vi "Tx Channel Config Page.vi"(8 "error in (no error)":errorcluster, 11 "Node Ptr":T1 format="%.0x") -> (0 "error out":errorcluster)   [LabVIEW 2019, in "UDP-Custom-Device System Explorer.lvlib"]
uses:
  UDP-Custom-Device System Explorer.lvlib
  <vilib>/NI VeriStand/Custom Device API/Custom Device Item Ref.ctl
  Shared/Constants.vi
  <vilib>/NI VeriStand/Custom Device API/Set Item Property (Boolean).vi
  <vilib>/NI VeriStand/Custom Device API/Set Item Property (U32).vi
  <vilib>/NI VeriStand/Custom Device API/Custom Device API.lvlib
  Property Accessors/Shared Channel Accessors.lvlib
  <vilib>/NI VeriStand/Custom Device Tools/Custom Device Utility Library/Custom Device Utility Library.lvlib
  Shared/UDP-Custom-Device Shared.lvlib
panel:
  in  "Append To Channels":bool
  in  "Instances To Create":u32=1 min=1 step=1
  out "Imported Channel Configuration":i32[](listbox) caption="Channels"
  in  "Channel Configuration File":path
  in  "Description":string
  out "Name":string
  in  "SHDocVw.IWebBrowser":refnum<k7>(container)
  in  "General Header":cluster{"Section Name":string}={"Section Name"="Channel Configuration"}
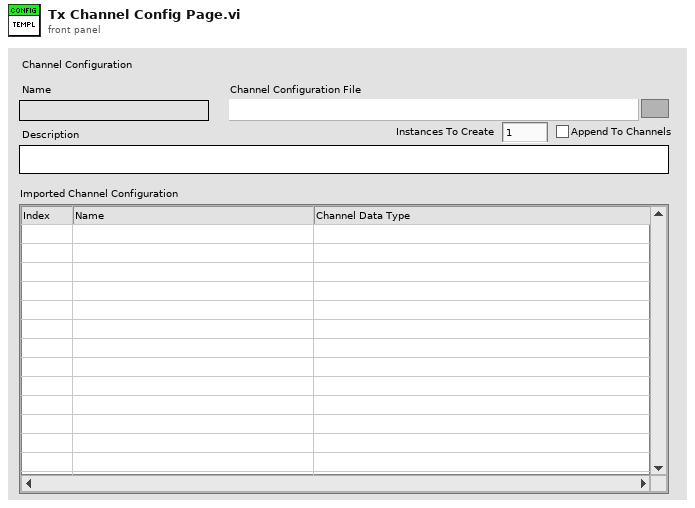
[diagram p1: front panel]
types:
  T1 = typedef "Custom Device API.lvlib/Custom Device Item Ref.ctl" = u64
  T2 = typedef "Custom Device API.lvlib/Custom Device Commands.ctl" = enum16{"Default", "Item renamed", "Shutdown", "Dynamic button pressed"}
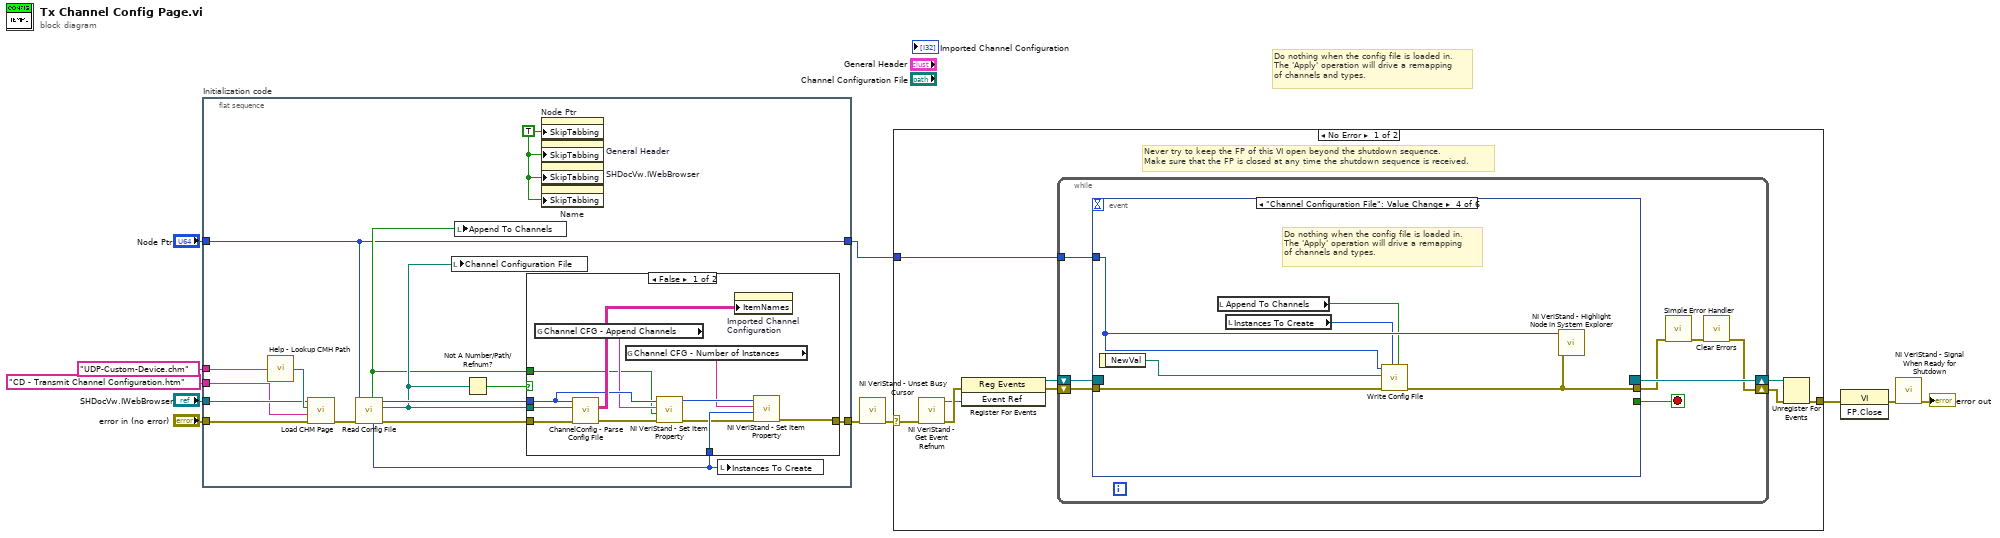
[diagram p0: block diagram]
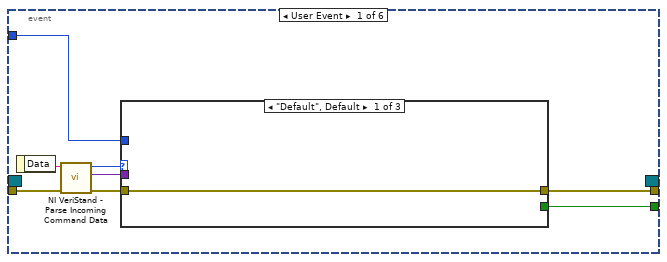
[diagram p3: hidden frame]
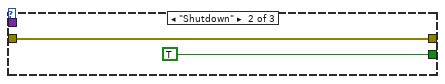
[diagram p4: hidden frame]
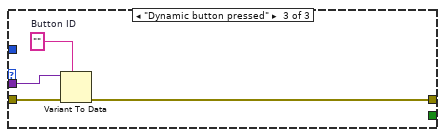
[diagram p5: hidden frame]
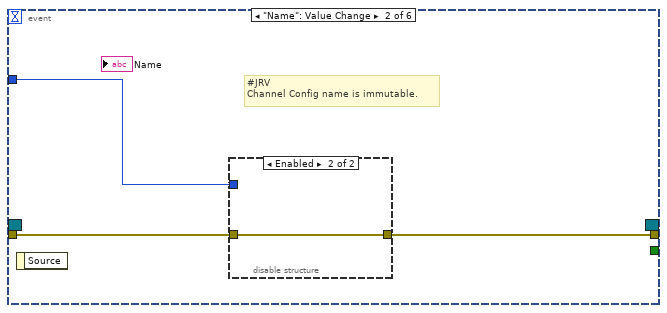
[diagram p6: hidden frame]
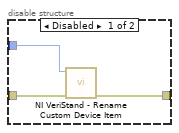
[diagram p7: hidden frame]
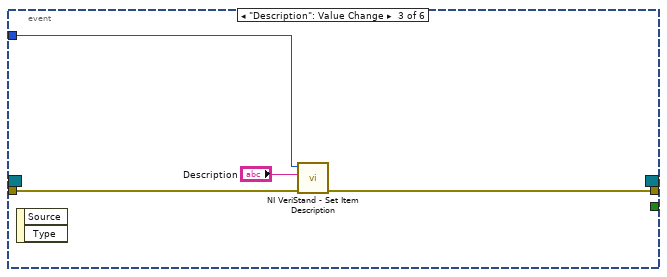
[diagram p8: hidden frame]
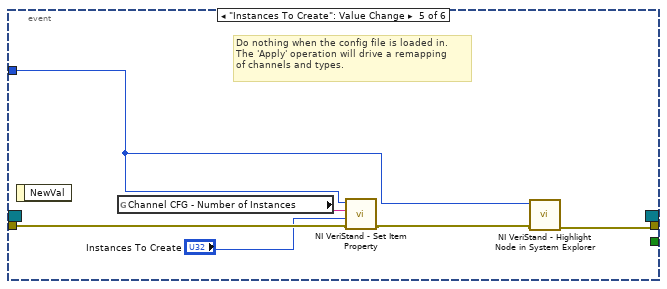
[diagram p9: hidden frame]
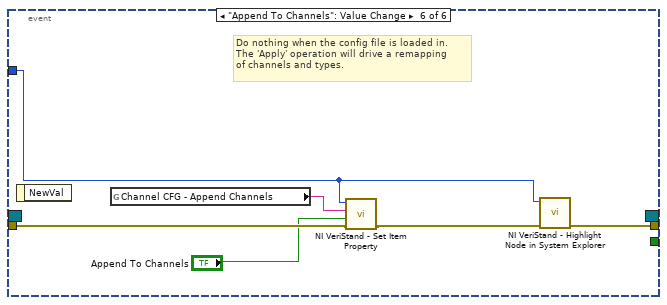
[diagram p10: hidden frame]
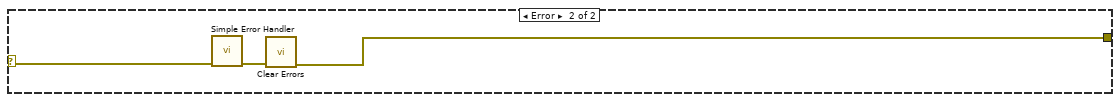
[diagram p11: hidden frame]
diagram:
  # "Do nothing when the config file is loaded in.\nThe 'Apply' operation will drive a remapping\nof channels and types."
  n1 = flat-sequence "Initialization code" {
    tunnel: "error in (no error)" -> [w25]
    tunnel: "Node Ptr" -> [w12]
    tunnel: [w16] -> w7
    tunnel: [w12] -> w4
    tunnel: "SHDocVw.IWebBrowser" -> [w24]
    tunnel: "CD - Transmit Channel Configuration.htm" ("CD_CHM_Section") -> [w22]
    tunnel: "UDP-Custom-Device.chm" ("CD_CHM_FileName") -> [w23]
    frame #0 {
      w15 = TRUE ("Skip When Tabbing")
      n2 = call "Help - Lookup CMH Path.vi"("Main CMH File"=w23) -> ("Compiled CMH Path"=w26:path)
      n3 = call <vilib>:"Load CHM Page.vi"("error in (no error)"=w25, "HTML File"=w22, "Compiled CHM Path"=w26, "Web Browser Reference"=w24) -> ("error out"=w21:errorcluster)  [unwired: 7 in]
      n4 = call "Read Config File.vi"("error in (no error)"=w21, "Node Ptr"=w12) -> ("error out"=w20:errorcluster, "Config File"=w17:path, "Node Ptr out"=w18:T1, "NumberOfInstances"=w13:u32, "AppendToChannels"=w14:bool)  [unwired: 5 in]
      n5 = local write "Channel Configuration File"(w17) -> ()
      n6 = local write "Append To Channels"(w14) -> ()
      n7 = Not A Number/Path/Refnum?(number/path/refnum=w17) -> (NaN/Path/Refnum?=w19:bool)
      n8 = case shown="False" w19 {
        tunnel: w20 -> [w38 w39]
        tunnel: w18 -> [w34 _]
        tunnel: w17 -> [w37 _]
        tunnel: [w27 w39] -> w16
        tunnel: w14 -> [w31 _]
        tunnel: w13 -> [w30 _]
        frame False {
          n9 = global read "Constants.vi" "Channel CFG - Append Channels"() -> (w33:string)
          n10 = call "ChannelConfig - Parse Config File.vi"("error in (no error)"=w38, "Config Path"=w37, "Node Ptr"=w34) -> ("error out"=w29:errorcluster, "Channel Configuration"=w36:string[][])  [unwired: 6 in, 1 out]
          n11 = global read "Constants.vi" "Channel CFG - Number of Instances"() -> (w32:string)
          n12 = call-poly <vilib>:"NI VeriStand - Set Item Property.vi"("error in (no error)"=w29, "Value"=w31, "Property Name"=w33, "Item Ref in"=w34) -> ("error out"=w28:errorcluster, "Item Ref out"=w35:T1)  [unwired: 5 in, 1 out]
          n13 = property on="Imported Channel Configuration" class="MCListbox (strict)"("ItemNames"=w36) -> ()  [unwired: 2 in, 2 out]
          n14 = call-poly <vilib>:"NI VeriStand - Set Item Property.vi"("error in (no error)"=w28, "Value"=w30, "Property Name"=w32, "Item Ref in"=w35) -> ("error out"=w27:errorcluster)  [unwired: 5 in, 2 out]
        }
        frame True {
        }
      }
      n15 = property on="Node Ptr" class="DigNum (strict)"("SkipTabbing"=w15) -> ()  [unwired: 2 in, 2 out]
      n16 = property on="General Header" class="Clust (strict)"("SkipTabbing"=w15) -> ()  [unwired: 2 in, 2 out]
      n17 = property on="SHDocVw.IWebBrowser" class="AXCont"("SkipTabbing"=w15) -> ()  [unwired: 2 in, 2 out]
      n18 = property on="Name" class="Str"("SkipTabbing"=w15) -> ()  [unwired: 2 in, 2 out]
      n19 = local write "Instances To Create"(w13) -> ()
    }
  }
  n20 = call <vilib>:"NI VeriStand - Unset Busy Cursor.vi"("error in (no error)"=w7) -> ("error out"=w6:errorcluster)  [unwired: 10 out]
  n21 = case shown="No Error" w6 {
    selector: w6 -> [w40 w103]
    tunnel: [w45 w101] -> w11
    tunnel: w4 -> [w41 _]
    frame No Error {
      # "Never try to keep the FP of this VI open beyond the shutdown sequence.\nMake sure that the FP is closed at any time the shutdown sequence is received."
      n22 = call <vilib>:"NI VeriStand - Get Event Refnum.vi"("error in (no error)"=w40) -> ("error out"=w48:errorcluster, "Event Ref"=w44:refnum<user-event>)  [unwired: 9 out]
      n23 = register-events(error in=w48, w44) -> (reference out=w42:refnum<event-registration>, error out=w43:errorcluster)  [unwired: 1 in]
      n24 = while {
        tunnel: w41 -> [w52]
        shift-right: [w49] -> w46
        shift-left: w43 -> [w55]
        shift-right: [w56] -> w47
        shift-left: w42 -> [w54]
        stop <- w53 stop-if-true
        n25 = event shown="[3] \"Channel Configuration File\": Value Change" {
          selector: w54 -> [_ _ _ _ _ _]
          dyn-events: [_ _ _ _ _ _] -> w56
          timeout: _ -> [_ _ _ _ _ _]
          tunnel: w55 -> [w64 w74 w82 w86 w94 w100]
          tunnel: [w60 _ _ _ _ _] -> w53
          tunnel: [w59 w72 w79 w85 w90 w97] -> w51
          tunnel: w52 -> [w58 w73 w81 w88 w91 w96]
          event User Event {
            n26 = event-data() -> ("Data"=w63:string)  [unwired: 1 out]
            n27 = call <vilib>:"NI VeriStand - Parse Incoming Command Data.vi"("error in (no error)"=w64, "Incoming data"=w63) -> ("error out"=w62:errorcluster, "Outgoing data"=w57:variant, "Action"=w61:T2)  [unwired: 7 out]
            n28 = case shown="\"Default\", Default" w61 {
              tunnel: w62 -> [w65 w66 w71]
              tunnel: [_ TRUE _] -> w60
              tunnel: [w65 w66 w68] -> w59
              tunnel: w58 -> [_ _ _]
              tunnel: w57 -> [_ _ w70]
              frame "Default", Default {
              }
              frame "Shutdown" {
              }
              frame "Dynamic button pressed" {
                w69 = ""  # Button ID
                n29 = Variant To Data(error in=w71, type=w69, Variant=w70) -> (error out=w68:errorcluster)  [unwired: 1 out]
              }
            }
          }
          event "Name": Value Change {
            # "#JRV\nChannel Config name is immutable."
            n30 = event-data() -> ()  [unwired: 2 out]
            n31 = disable-structure shown="Enabled" {
              disable-tunnel: w74 -> [w77 w78]
              disable-tunnel: w73 -> [w76 _]
              disable-tunnel: [w75 w78] -> w72
              frame Disabled {
                n32 = call <vilib>:"NI VeriStand - Rename Custom Device Item.vi"("error in (no error)"=w77, "Item Ref in"=w76) -> ("error out"=w75:errorcluster)  [unwired: 7 in, 2 out]
              }
              frame Enabled {
              }
            }
          }
          event "Description": Value Change {
            n33 = event-data() -> ()  [unwired: 3 out]
            n34 = call <vilib>:"NI VeriStand - Set Item Description.vi"("error in (no error)"=w82, "Description"="Description", "Item Ref in"=w81) -> ("error out"=w79:errorcluster)  [unwired: 6 in, 2 out]
          }
          event "Channel Configuration File": Value Change {
            # "Do nothing when the config file is loaded in.\nThe 'Apply' operation will drive a remapping\nof channels and types."
            n35 = event-data() -> ("NewVal"=w87:path)  [unwired: 1 out]
            n36 = local read "Append To Channels"() -> (w84:bool)
            n37 = local read "Instances To Create"() -> (w83:u32)
            n38 = call "Write Config File.vi"("Append To Channels"=w84, "Instances To Create"=w83, "error in (no error)"=w86, "Config File"=w87, "Node Ptr"=w88) -> ("error out"=w85:errorcluster)  [unwired: 5 in, 1 out]
            n39 = call <vilib>:"NI VeriStand - Highlight Node in System Explorer.vi"("error in (no error)"=w85, "Item Ref in"=w88) -> ()  [unwired: 8 in, 2 out]
          }
          event "Instances To Create": Value Change {
            # "Do nothing when the config file is loaded in.\nThe 'Apply' operation will drive a remapping\nof channels and types."
            n40 = event-data() -> ()  [unwired: 2 out]
            n41 = global read "Constants.vi" "Channel CFG - Number of Instances"() -> (w93:string)
            n42 = call-poly <vilib>:"NI VeriStand - Set Item Property.vi"("error in (no error)"=w94, "Value"="Instances To Create", "Property Name"=w93, "Item Ref in"=w91) -> ("error out"=w92:errorcluster)  [unwired: 5 in, 2 out]
            n43 = call <vilib>:"NI VeriStand - Highlight Node in System Explorer.vi"("error in (no error)"=w92, "Item Ref in"=w91) -> ("error out"=w90:errorcluster)  [unwired: 8 in, 1 out]
          }
          event "Append To Channels": Value Change {
            # "Do nothing when the config file is loaded in.\nThe 'Apply' operation will drive a remapping\nof channels and types."
            n44 = event-data() -> ()  [unwired: 2 out]
            n45 = global read "Constants.vi" "Channel CFG - Append Channels"() -> (w99:string)
            n46 = call-poly <vilib>:"NI VeriStand - Set Item Property.vi"("error in (no error)"=w100, "Value"="Append To Channels", "Property Name"=w99, "Item Ref in"=w96) -> ("error out"=w98:errorcluster)  [unwired: 5 in, 2 out]
            n47 = call <vilib>:"NI VeriStand - Highlight Node in System Explorer.vi"("error in (no error)"=w98, "Item Ref in"=w96) -> ("error out"=w97:errorcluster)  [unwired: 8 in, 1 out]
          }
        }
        n48 = call <vilib>:"Simple Error Handler.vi"("error in (no error)"=w51) -> ("error out"=w50:errorcluster)  [unwired: 1 in, 7 out]
        n49 = call <vilib>:"Clear Errors.vi"("error in (no error)"=w50) -> ("error out"=w49:errorcluster)  [unwired: 1 in, 5 out]
      }
      n50 = Unregister For Events(event registration refnum=w47, error in=w46) -> (error out=w45:errorcluster)
    }
    frame Error {
      n51 = call <vilib>:"Simple Error Handler.vi"("error in (no error)"=w103) -> ("error out"=w102:errorcluster)  [unwired: 1 in, 7 out]
      n52 = call <vilib>:"Clear Errors.vi"("error in (no error)"=w102) -> ("error out"=w101:errorcluster)  [unwired: 1 in, 5 out]
    }
  }
  n53 = invoke class="VI" method="FP.Close"(error in=w11) -> (error out=w10:errorcluster)  [unwired: 2 in, 2 out]
  n54 = call <vilib>:"NI VeriStand - Signal When Ready for Shutdown.vi"("error in (no error)"=w10) -> ("error out"=→"error out":errorcluster)  [unwired: 10 out]
